vi "AccessLog写入.vi"(11 "Log":string) -> ()   [LabVIEW 2016, in "斯坦道总氮.lvlib"]
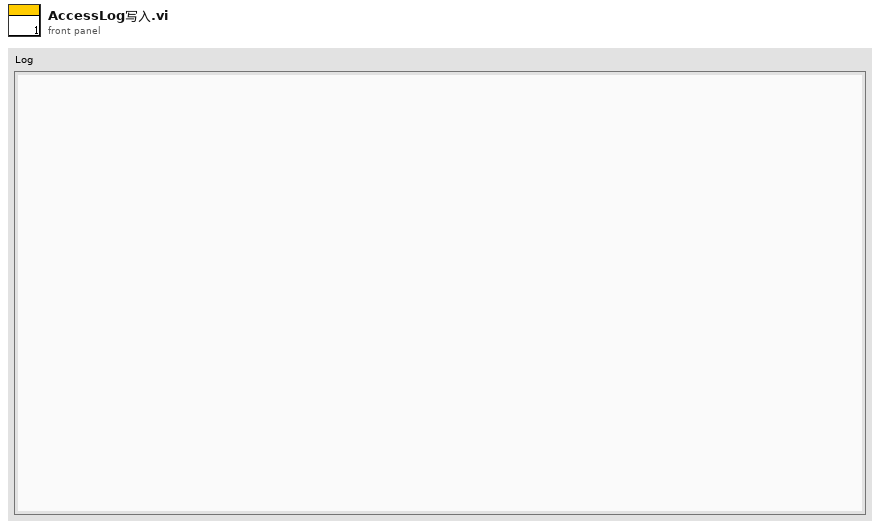
[diagram p1: front panel]
types:
  T1 = enum16{"open", "replace", "create", "open or create", "replace or create", "replace or create with confirmation"}
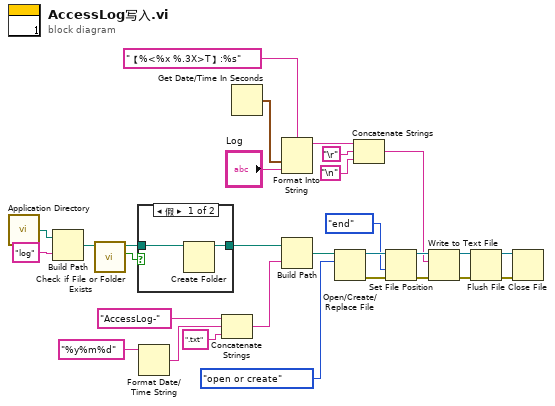
[diagram p0: block diagram]
diagram:
  n1 = call <vilib>:"Application Directory.vi"() -> ("Application Directory"=w7:path)
  n2 = Build Path(base path=w7, name or relative path="log" ("名称或相对路径")) -> (appended path=w5:path)
  n3 = call <vilib>:"Check if File or Folder Exists.vi"("path"=w5) -> ("file or folder exists?"=w20:bool, "dup path"=w19:path)  [unwired: 8 in, 1 out]
  n4 = case shown="假" w20 {
    tunnel: w19 -> [w31 w32]
    tunnel: [w30 w32] -> w18
    frame False {
      n5 = Create Folder(path (use dialog)=w31) -> (created path=w30:path)  [unwired: 2 in, 2 out]
    }
    frame True {
    }
  }
  n6 = Format Date/Time String(time format string (%c)="%y%m%d" ("时间格式字符串(%c)")) -> (date/time string=w16:string)  [unwired: 2 in]
  n7 = Concatenate Strings("AccessLog-" ("字符串"), w16, ".txt" ("字符串")) -> (w15:string)
  n8 = Get Date/Time In Seconds() -> (seconds since 1Jan1904=w28:timestamp)
  n9 = Format Into String(format string="【%<%x %.3X>T】:%s" ("格式字符串"), w28, "Log") -> (resulting string=w27:string)  [unwired: 2 in, 1 out]
  n10 = Build Path(base path=w18, name or relative path=w15) -> (appended path=w14:path)
  n11 = Open/Create/Replace File(file path (use dialog)=w14, operation (0:open)=T1."open or create" ("操作(0:open)")) -> (refnum out=w22:refnum<file>, error out=w24:errorcluster)  [unwired: 4 in, 1 out]
  n12 = Concatenate Strings(w27, "\r", "\n") -> (w3:string)
  n13 = Set File Position(refnum=w22, from (0:start)=enum16{"start", "end", "current"}."end" ("自（0:起始）"), error in=w24) -> (refnum out=w23:refnum<file>, error out=w25:errorcluster)  [unwired: 1 in]
  n14 = Write to Text File(file (use dialog)=w23, text=w3, error in=w25) -> (refnum out=w10:refnum<file>, error out=w9:errorcluster)  [unwired: 1 in, 1 out]
  n15 = Flush File(refnum=w10, error in=w9) -> (refnum out=w12:refnum<file>, error out=w11:errorcluster)
  n16 = Close File(refnum=w12, error in=w11) -> ()  [unwired: 2 out]
